vi "Move.vi"(8 "error in (no error)":errorcluster, 9 "Absolute (T)":bool=TRUE, 10 "Point":refnum<class "Point.lvclass">, 11 "RoundRectangle in":refnum<class "RoundRectangle.lvclass">) -> (0 "error out":errorcluster, 3 "RoundRectangle out":refnum<class "RoundRectangle.lvclass">)   [LabVIEW 2021, in "Picture2D.lvlib" / "RoundRectangle.lvclass"]
uses:
  RoundRectangle.lvclass
  Rectangle/Rectangle.lvclass
  Point/Point.lvclass
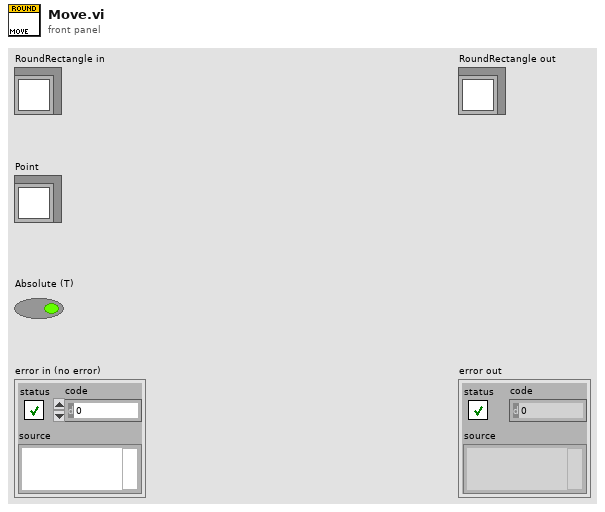
[diagram p1: front panel]
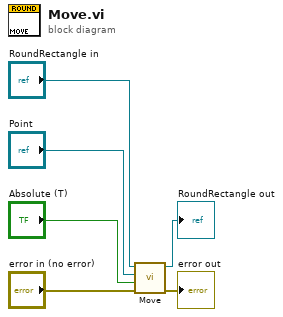
[diagram p0: block diagram]
diagram:
  n1 = call-parent "Move.vi"("error in (no error)"="error in (no error)", "Absolute (T)"="Absolute (T)", "Point"="Point", "Rectangle in"="RoundRectangle in") -> ("error out"=→"error out":errorcluster, "Rectangle out"=→"RoundRectangle out":refnum<class "RoundRectangle.lvclass">)  [unwired: 6 in]
